vi "compare r140 and libre.vi"() -> ()   [LabVIEW 2020]
uses:
  common/record_file_handler/VFH-VNA_File_Handler.lvlib
panel:
  out "s11''":cluster{"Frequency":dbl[], "S21_Imag":dbl[]}[](graph)
  out "s11":cluster{"Frequency":dbl[], "S21_Imag":dbl[]}[](graph)
  out "size(s) 2":i32
  out "size(s)":i32
  out "r140":string[](array[string])
  out "Libre":string[](array[string])
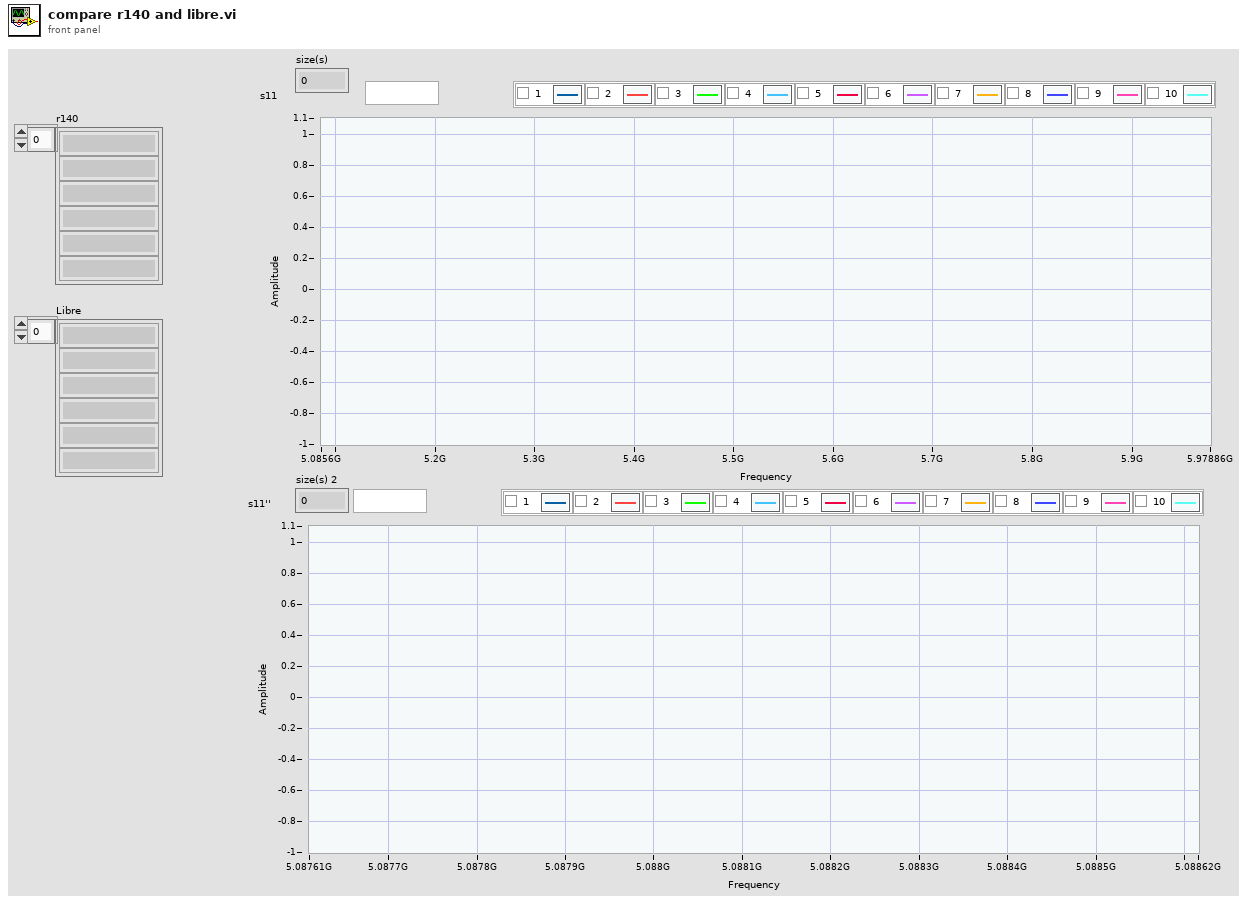
[diagram p1: front panel]
types:
  T1 = typedef "VFH-VNA_File_Handler.lvlib/VFH-file_cluster-NanoVNA.ctl" = cluster{"Frequency":dbl[], "S11_Real":dbl[], "S11_Imag":dbl[], "S21_Real":dbl[], "S21_Imag":dbl[], "S12_Real":dbl[], "S12_Imag":dbl[], "S22_Real":dbl[], "S22_Imag":dbl[]}
  T2 = typedef "VFH-VNA_File_Handler.lvlib/VFH-file_cluster-r140.ctl" = cluster{"Frequency":dbl[], "Permativity'":dbl[], "Permativity''":dbl[], "Q [S/m]":dbl[], "Tan":dbl[], "Reflection R":dbl[], "Reflection I":dbl[]}
  T3 = cluster{"Frequency":dbl[], "Reflection R":dbl[]}[]
  T4 = cluster{"Frequency":dbl[], "Reflection I":dbl[]}[]
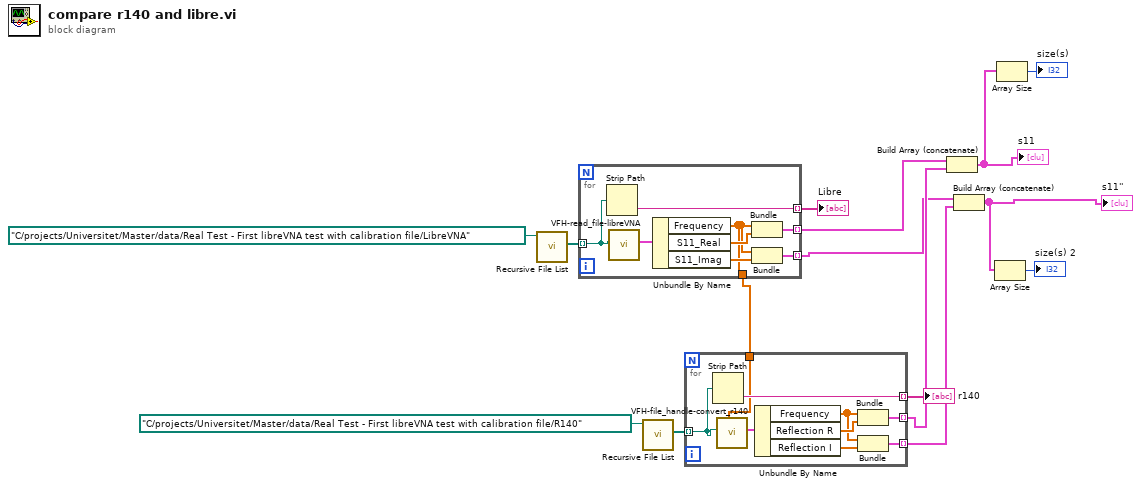
[diagram p0: block diagram]
diagram:
  n1 = call <vilib>:"Recursive File List.vi"("Folder Path"=path "C:/projects/Universitet/Master/data/Real Test - First libreVNA test with calibration file/LibreVNA" ("base path")) -> ("All Files in Dir"=w14:path[])  [unwired: 6 in, 4 out]
  n2 = for {
    tunnel: [w21] -> w9 mode=indexing
    tunnel: [w20] -> w6 mode=indexing
    tunnel: w14 -> [w17] mode=indexing
    tunnel: [w19] -> w13 mode=indexing
    tunnel: [w16] -> w3
    n3 = Strip Path(path=w17) -> (name=w19:string)  [unwired: 1 out]
    n4 = call "VFH-read_file-libreVNA.vi"("file path (dialog if empty)"=w17) -> ("output cluster"=w18:T1)  [unwired: 9 in, 1 out]
    n5 = Unbundle By Name(w18) -> ("Frequency"=w16:dbl[], "S11_Real"=w23:dbl[], "S11_Imag"=w22:dbl[])
    n6 = Bundle("Frequency"=w16, "S11_Real"=w23) -> (w21:cluster{"Frequency":dbl[], "S11_Real":dbl[]})  [unwired: 1 in]
    n7 = Bundle("Frequency"=w16, "S11_Imag"=w22) -> (w20:cluster{"Frequency":dbl[], "S11_Imag":dbl[]})  [unwired: 1 in]
  }
  "Libre" <- w13
  n8 = call <vilib>:"Recursive File List.vi"("Folder Path"=path "C:/projects/Universitet/Master/data/Real Test - First libreVNA test with calibration file/R140" ("base path")) -> ("All Files in Dir"=w11:path[])  [unwired: 6 in, 4 out]
  n9 = for {
    tunnel: [w29] -> w8 mode=indexing
    tunnel: [w28] -> w7 mode=indexing
    tunnel: w11 -> [w26] mode=indexing
    tunnel: [w27] -> w10 mode=indexing
    tunnel: w3 -> [w24]
    n10 = Strip Path(path=w26) -> (name=w27:string)  [unwired: 1 out]
    n11 = call "VFH-file_handle-convert_r140.vi"("Xi"=w24, "file path (dialog if empty)"=w26) -> ("Handled data"=w25:T2)  [unwired: 9 in]
    n12 = Unbundle By Name(w25) -> ("Frequency"=w30:dbl[], "Reflection R"=w32:dbl[], "Reflection I"=w31:dbl[])
    n13 = Bundle("Frequency"=w30, "Reflection R"=w32) -> (w29:cluster{"Frequency":dbl[], "Reflection R":dbl[]})  [unwired: 1 in]
    n14 = Bundle("Frequency"=w30, "Reflection I"=w31) -> (w28:cluster{"Frequency":dbl[], "Reflection I":dbl[]})  [unwired: 1 in]
  }
  "r140" <- w10
  n15 = Build Array (concatenate)(w9, w8) -> (w1:T3)
  "s11" <- w1
  n16 = Build Array (concatenate)(w6, w7) -> (w2:T4)
  "s11''" <- w2
  n17 = Array Size(array=w2) -> (size(s)=→"size(s) 2":i32)
  n18 = Array Size(array=w1) -> (size(s)=→"size(s)":i32)
